vi "GetSlideDigits.vi"(6 "error in":errorcluster, 9 "Scale":refnum<class "Scale.lvclass">) -> (0 "error out":errorcluster, 3 "Scale out":refnum<class "Scale.lvclass">, 4 "digits":i32)   [LabVIEW 2014, in "PythonConverter_GUI.lvclass"]
uses:
  PythonConverter_GUI.lvclass
  VI Interpreter/Classes/Scale/Scale.lvclass
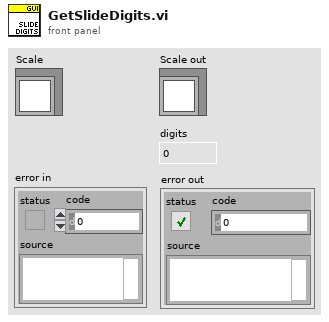
[diagram p1: front panel]
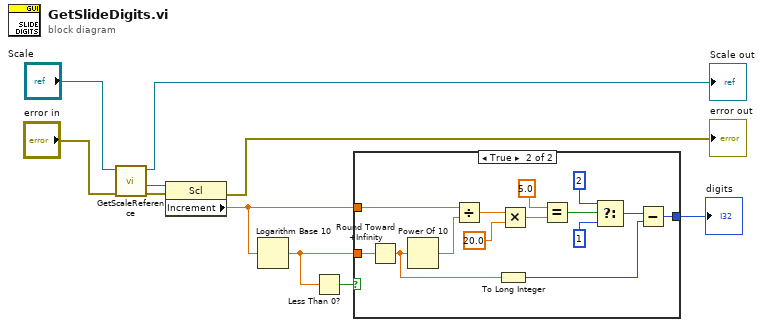
[diagram p0: block diagram]
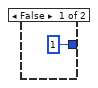
[diagram p2: hidden frame]
diagram:
  n1 = call "GetScaleReference.vi"("error in"="error in", "Scale in"="Scale") -> ("error out"=w7:errorcluster, "scale reference"=w8:refnum<vi>, "Scale out"=→"Scale out":refnum<class "Scale.lvclass">)  [unwired: 7 in]
  n2 = property on="Property Node" class="Scl"(reference=w8, error in=w7) -> (error out=→"error out":errorcluster, "Increment"=w3:dbl)  [unwired: 1 out]
  n3 = Logarithm Base 10(1:w3) -> (0:w5:dbl)
  n4 = Less Than 0?(x=w5) -> (x < 0?=w4:bool)
  n5 = case shown="True" w4 {
    tunnel: w5 -> [_ w25]
    tunnel: w3 -> [_ w24]
    tunnel: [1 w12] -> w6
    frame False {
    }
    frame True {
      n6 = Round Toward +Infinity(x=w25) -> (ceil(x): smallest int >= x=w14:dbl)
      n7 = Power Of 10(x=w14) -> (10^x=w23:dbl)
      n8 = Divide(x=w24, y=w23) -> (x/y=w21:dbl)
      n9 = To Long Integer(number=w14) -> (32bit integer=w13:i32)
      n10 = Multiply(x=w21, y=20.0) -> (x*y=w20:dbl)
      n11 = Equal?(x=5.0, y=w20) -> (x = y?=w18:bool)
      n12 = Select(t=2, s=w18, f=1) -> (s? t:f=w15:i32)
      n13 = Subtract(x=w15, y=w13) -> (x-y=w12:i32)
    }
  }
  "digits" <- w6
